vi "Telnet Registry.vi"(7 "function (get data)":T2(ring)=enum."get data", 8 "error in (no error)":errorcluster, 10 "object data in":T3, 11 "object":T1) -> (0 "error out":errorcluster, 1 "objects":T1[](array[typedef]), 2 "object data":T3, 3 "object out":T1, 4 "valid index?":bool)   [LabVIEW 2014]
doc: "Keeps track of data associated with an object. The function parameter is used to operate on objects.\n\n* reset: Destroys and removes all objects from the registry\n* register: Adds an object to registry (returns error if object is already registered)\n* get data: Returns the data associated with an object (returns error if object is not registered)\n* set data: Sets the data associated with an object (returns error if object is not registered)\n* unregister: Destroys and removes the object from the registry (returns error if object is not registered)\n* get objects: Returns all registered objects"
uses:
  Telnet Session.ctl
  Telnet Connection Data.ctl
  Semaphore RefNum.ctl
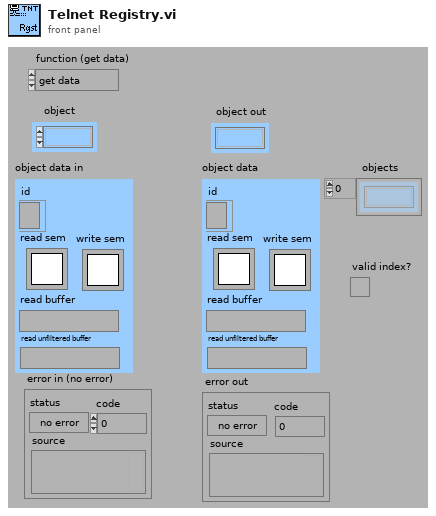
[diagram p1: front panel]
types:
  T1 = typedef "Telnet Session.ctl" = refnum<k1>
  T2 = enum16{"reset", "register", "get data", "set data", "unregister", "test", "get objects"}
  T3 = typedef "Telnet Connection Data.ctl" = cluster{"id":refnum<k5>, "read sem":T4, "write sem":T4, "read buffer":string, "read unfiltered buffer":string}
  T4 = typedef "Semaphore RefNum.ctl" = refnum<k1>
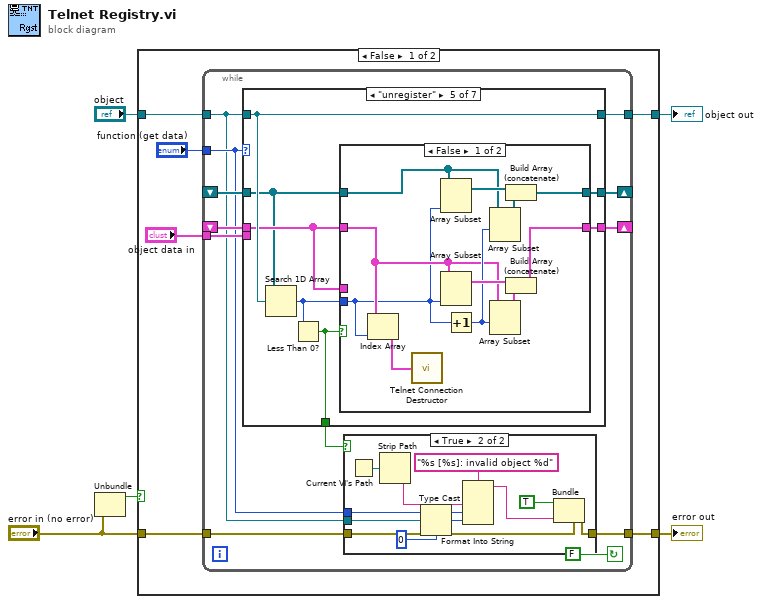
[diagram p0: block diagram]
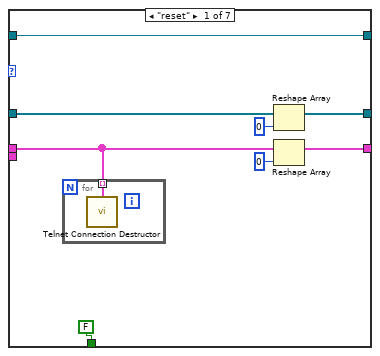
[diagram p3: hidden frame]
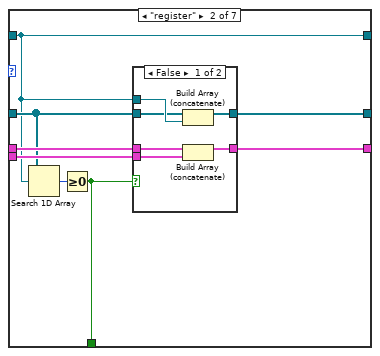
[diagram p4: hidden frame]
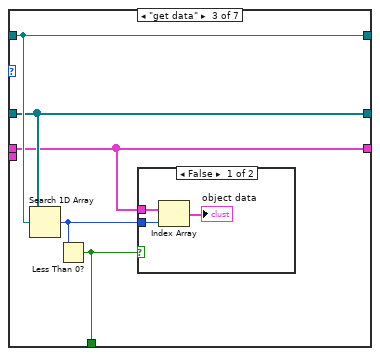
[diagram p6: hidden frame]
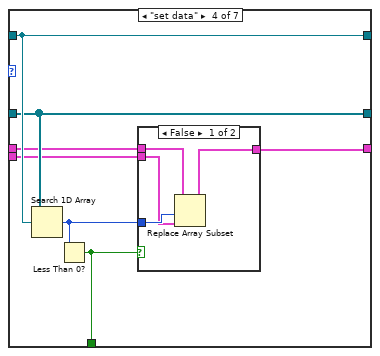
[diagram p8: hidden frame]
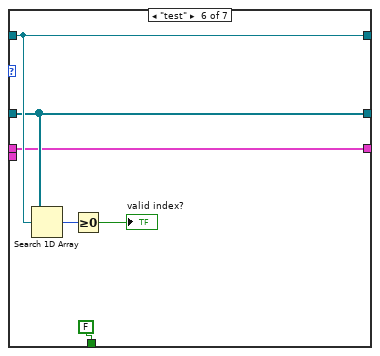
[diagram p11: hidden frame]
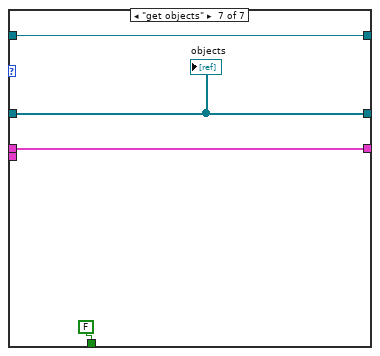
[diagram p12: hidden frame]
diagram:
  n1 = Unbundle("error in (no error)") -> ("status"=w3:bool)  [unwired: 2 out]
  n2 = case shown="False" w3 {
    tunnel: "error in (no error)" -> [w11 w112]
    tunnel: [w8 w111] -> w5
    tunnel: [w7 w112] -> w2
    tunnel: "object" -> [w6 w111]
    frame False {
      n3 = while {
        tunnel: [w13] -> w7
        tunnel: w11 -> [w14]
        tunnel: "object data in" -> [w17]
        tunnel: "function (get data)" -> [w16]
        tunnel: [w19] -> w8
        tunnel: w6 -> [w15]
        shift-left: _ -> [w21]
        shift-right: [w20] -> _
        shift-left: _ -> [w23]
        shift-right: [w22] -> _
        stop <- FALSE continue-if-true
        n4 = case shown="\"unregister\"" w16 {
          tunnel: w23 -> [w39 w47 w64 w74 w84 w104 w110]
          tunnel: w15 -> [w37 w46 w65 w75 w87 w106 w108]
          tunnel: [w37 w46 w65 w75 w87 w106 w108] -> w19
          tunnel: [w38 w52 w64 w74 w83 w104 w110] -> w22
          tunnel: [w42 w50 w62 w71 w82 w103 w109] -> w20
          tunnel: w21 -> [w43 w51 w62 w72 w85 w103 w109]
          tunnel: w17 -> [_ w49 _ w70 _ _ _]
          tunnel: [FALSE w45 w61 w69 w81 FALSE FALSE] -> w18
          frame "reset" {
            n5 = for {
              tunnel: w43 -> [w44] mode=indexing
              n6 = call "Telnet Connection Destructor.vi"("object data in"=w44) -> ()
            }
            n7 = Reshape Array(w39, 0) -> (w38:T1[])
            n8 = Reshape Array(w43, 0) -> (w42:T3[])
          }
          frame "register" {
            n9 = Search 1D Array(1D array=w47, element=w46) -> (index of element=w48:i32)  [unwired: 1 in]
            n10 = Greater Or Equal To 0?(x=w48) -> (x >= 0?=w45:bool)
            n11 = case shown="False" w45 {
              tunnel: w46 -> [w58 _]
              tunnel: w47 -> [w57 w60]
              tunnel: w49 -> [w56 _]
              tunnel: [w55 w59] -> w50
              tunnel: w51 -> [w54 w59]
              tunnel: [w53 w60] -> w52
              frame False {
                n12 = Build Array (concatenate)(w57, w58) -> (w53:T1[])
                n13 = Build Array (concatenate)(w54, w56) -> (w55:T3[])
              }
              frame True {
              }
            }
          }
          frame "get data" {
            n14 = Search 1D Array(1D array=w64, element=w65) -> (index of element=w63:i32)  [unwired: 1 in]
            n15 = Less Than 0?(x=w63) -> (x < 0?=w61:bool)
            n16 = case shown="False" w61 {
              tunnel: w63 -> [w68 _]
              tunnel: w62 -> [w67 _]
              frame False {
                n17 = Index Array(array=w67, index=w68) -> (element=→"object data":T3)
              }
              frame True {
              }
            }
          }
          frame "set data" {
            n18 = Search 1D Array(1D array=w74, element=w75) -> (index of element=w73:i32)  [unwired: 1 in]
            n19 = Less Than 0?(x=w73) -> (x < 0?=w69:bool)
            n20 = case shown="False" w69 {
              tunnel: w73 -> [w79 _]
              tunnel: w72 -> [w78 w80]
              tunnel: w70 -> [w77 _]
              tunnel: [w76 w80] -> w71
              frame False {
                n21 = Replace Array Subset(array=w78, new element=w77, index=w79) -> (w76:T3[])
              }
              frame True {
              }
            }
          }
          frame "unregister" {
            n22 = Search 1D Array(1D array=w84, element=w87) -> (index of element=w86:i32)  [unwired: 1 in]
            n23 = Less Than 0?(x=w86) -> (x < 0?=w81:bool)
            n24 = case shown="False" w81 {
              tunnel: w86 -> [w89 _]
              tunnel: w85 -> [_ _]
              tunnel: w85 -> [w90 w99]
              tunnel: w84 -> [w93 w100]
              tunnel: [w92 w100] -> w83
              tunnel: [w91 w99] -> w82
              frame False {
                n25 = Index Array(array=w90, index=w89) -> (element=w88:T3)
                n26 = call "Telnet Connection Destructor.vi"("object data in"=w88) -> ()
                n27 = Array Subset(array=w93, length=w89) -> (w95:T1[])  [unwired: 1 in]
                n28 = Array Subset(array=w90, length=w89) -> (w98:T3[])  [unwired: 1 in]
                n29 = Increment(x=w89) -> (x+1=w94:i32)
                n30 = Array Subset(array=w93, index=w94) -> (w96:T1[])  [unwired: 1 in]
                n31 = Array Subset(array=w90, index=w94) -> (w97:T3[])  [unwired: 1 in]
                n32 = Build Array (concatenate)(w95, w96) -> (w92:T1[])
                n33 = Build Array (concatenate)(w98, w97) -> (w91:T3[])
              }
              frame True {
              }
            }
          }
          frame "test" {
            n34 = Search 1D Array(1D array=w104, element=w106) -> (index of element=w105:i32)  [unwired: 1 in]
            n35 = Greater Or Equal To 0?(x=w105) -> (x >= 0?=→"valid index?":bool)
          }
          frame "get objects" {
            "objects" <- w110
          }
        }
        n36 = case shown="True" w18 {
          tunnel: w16 -> [_ w33]
          tunnel: w15 -> [_ w34]
          tunnel: w14 -> [w24 w32]
          tunnel: [w24 w29] -> w13
          frame False {
          }
          frame True {
            n37 = Current VI's Path() -> (path=w28:path)
            n38 = Strip Path(path=w28) -> (name=w27:string)  [unwired: 1 out]
            n39 = Type Cast(type=u32 0 ("object"), x=w34) -> (*(type *) &x=w26:u32)
            n40 = Format Into String(format string="%s [%s]: invalid object %d", w27, w33, w26) -> (resulting string=w31:string)  [unwired: 2 in, 1 out]
            n41 = Bundle(cluster=w32, "status"=TRUE, "source"=w31) -> (w29:errorcluster)  [unwired: 1 in]
          }
        }
      }
    }
    frame True {
    }
  }
  "object out" <- w5
  "error out" <- w2
